vi "WMS_DSP_System.vi"() -> ()   [LabVIEW 2019]
uses:
  <vilib>/Analysis/baseanly.llb/IIR Cascade Filter (DBL).vi
  <vilib>/Analysis/Matrix/Numeric/Conversions/Array To Matrix - RA.vi
  <vilib>/Utility/file.llb/Write Delimited Spreadsheet (DBL).vi
  <vilib>/Utility/file.llb/Read Delimited Spreadsheet (DBL).vi
  <vilib>/measure/NI_MABase.lvlib
  <vilib>/Analysis/NI_AALPro.lvlib
  <vilib>/Analysis/NI_AALBase.lvlib
  <vilib>/Analysis/Matrix/NI_Matrix.lvlib
  <vilib>/gmath/NI_Gmath.lvlib
panel:
  in  "STOP":bool
  in  "stop":bool
  in  "?":T1(tab)
  in  "?":T2(tab)
  out "2f/1f":cluster{dbl[], dbl[]}(graph)
  out "I_OUT":cluster{dbl[], dbl[]}(graph)
  out "First derivative":cluster{dbl[], dbl[]}(graph)
  out "Second derivative":cluster{dbl[], dbl[]}(graph)
  out "FFT of 1f":cluster{"f0":dbl, "df":dbl, "magnitude":dbl[]}(graph)
  out "FFT of 2f":cluster{"f0":dbl, "df":dbl, "magnitude":dbl[]}(graph)
  out "Charakterystyki absorpcyjne":cluster{dbl[], dbl[]}[](graph)
  in  "c [ppmv]":dbl=1.7
  in  "Load data from file":bool
  in  "Data path":path
  in  "l [m]":dbl=1000.0
  in  "c2 [ppmv]":dbl=7750.0
  in  "l2 [m]":dbl=1000.0
  in  "FWHM [nm]":dbl
  in  "ddelta_di [nm/mA]":dbl
  in  "dlambda [nm]":dbl
  in  "P0 [mW]":dbl
  in  "dP_di [mW/mA]":dbl
  in  "i_bias [mA]":dbl
  in  "Phase_IM_FM [rad]":dbl
  in  "lambda0 [nm]":dbl
  in  "m":dbl
  in  "f_ramp [Hz]":dbl
  in  "f [Hz]":dbl
  in  "Zapis parametrów do pliku":bool
  in  "Odczyt parametrów z pliku":bool
  in  "START":bool
  in  "l_s [m]":dbl=1.0
  in  "c_s [ppmv]":dbl=1.0
  in  "l_S2 [m]":dbl=1.0
  in  "c_s2 [ppmv]":dbl=1.0
  in  "f_LP1":dbl=800.0
  in  "f_LP2":dbl=1600.0
  in  "K":dbl=100.0
  in  "R":dbl=50.0
  in  "?":T3(tab)
  out "Signal from CH1":waveform(dbl)(graph)
  out "Signal from CH2":waveform(dbl)(graph)
  out "Signal 2f/1f":waveform(dbl)(graph)
  out "Averaged signal 2f/1f":waveform(dbl)(graph)
  out "1f":waveform(dbl)(graph)
  out "2f":waveform(dbl)(graph)
  in  "DAQ":bool
  in  "Liczba usrednien":dbl=10.0
  out "Licznik usrednien":dbl
  in  "f_LP2_DAQ":dbl=1600.0 format="%0.3f"
  in  "f_LP1_DAQ":dbl=800.0 format="%0.3f"
  in  "f_prob":dbl=100000.0
  in  "f_ref":dbl=10000.0
  in  "?":enum32{"Fitting", "2f/1f sym", "2f/1f pom"}(tab)
  out "Fitting":cluster{"t1":dbl[], "yi":dbl[]}[](graph)
  out "Simulation":waveform(dbl)(graph)
  out "Measurment":waveform(dbl)(graph)
  in  "START":bool
  out "c [ppmv]":dbl
  out "SE":dbl
  out "Searching":dbl(knob) scale=0.0..10.0
  out "Concentration":dbl(knob) scale=0.0..10.0
  in  "c1 [ppmv]":dbl
  in  "c2 [ppmv]":dbl=10.0
  out "c_po":dbl
  out "SE2":dbl
  in  "Precisiion [ppmv]":dbl=0.1
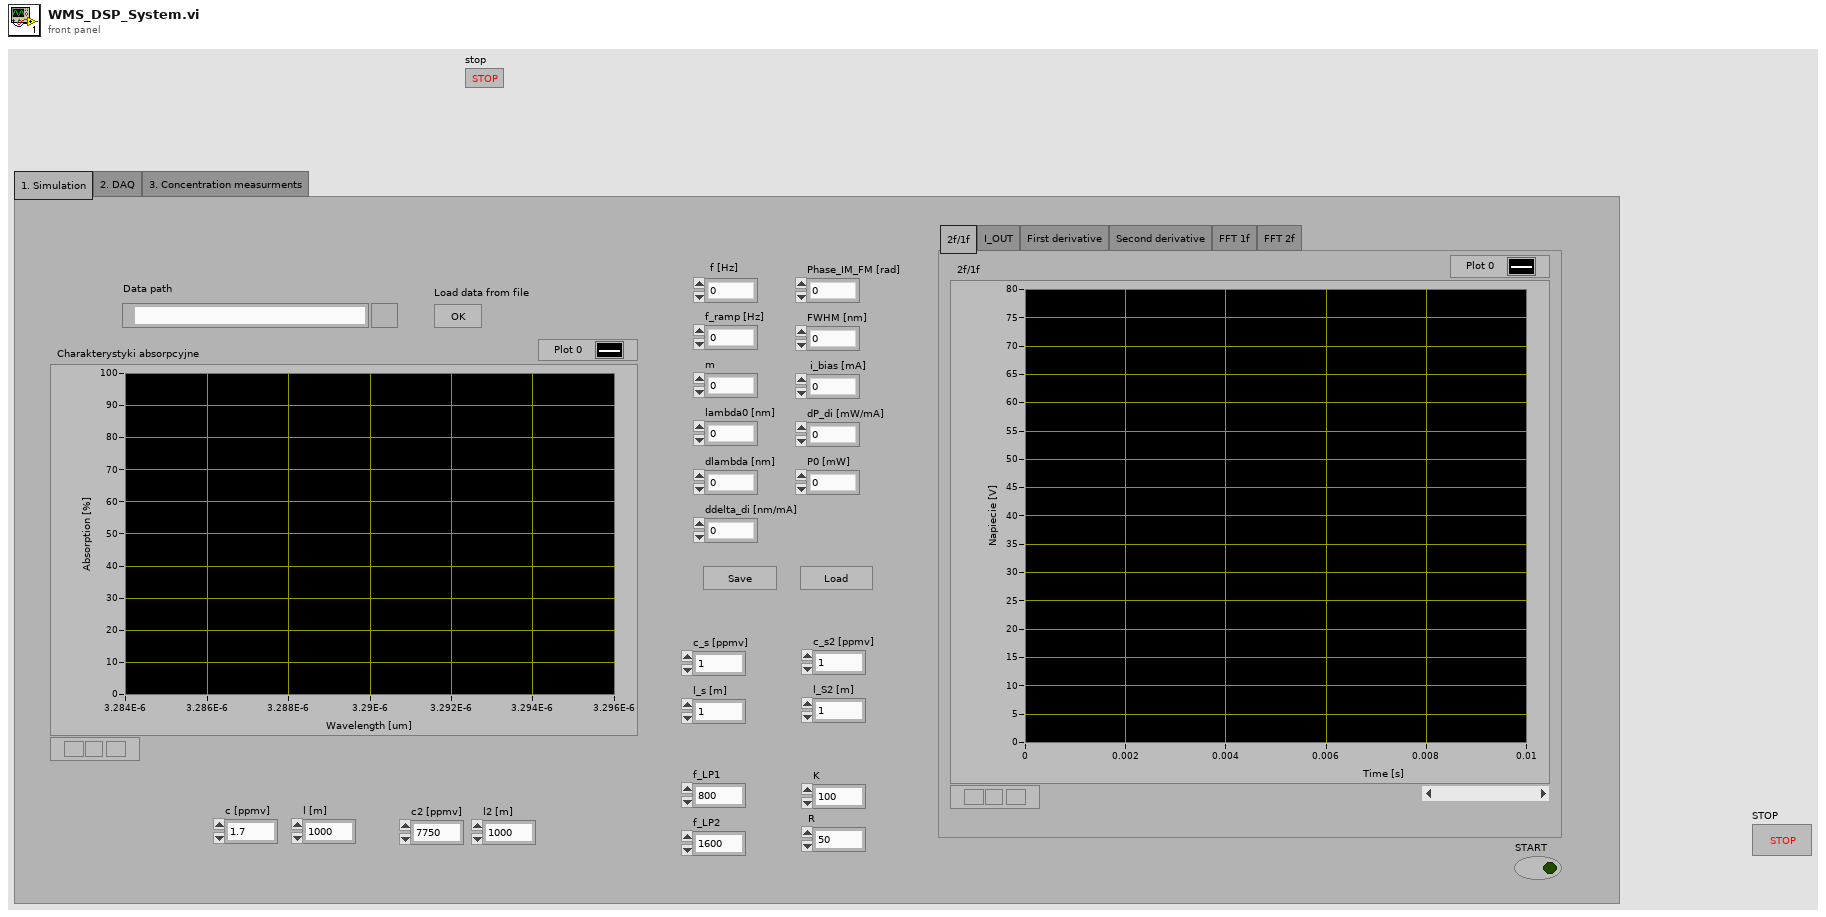
[diagram p1: front panel]
types:
  T1 = enum32{"1. Simulation", "2. DAQ", "3. Concentration measurments"}
  T2 = enum32{"2f/1f", "I_OUT", "First derivative", "Second derivative", "FFT 1f", "FFT 2f"}
  T3 = enum32{"Tor nr 1", "Tor nr 2", "2f/1f", "2f/1f usr", "1f me", "2f me"}
  T4 = cluster{"filter structure":enum32{"IIR 2nd Order", "IIR 4th Order"}, "Reverse Coefficients":dbl[], "Forward Coefficients":dbl[]}
  T5 = typedef "NI_Matrix.lvlib/RealMatrix.ctl" = dbl[][]
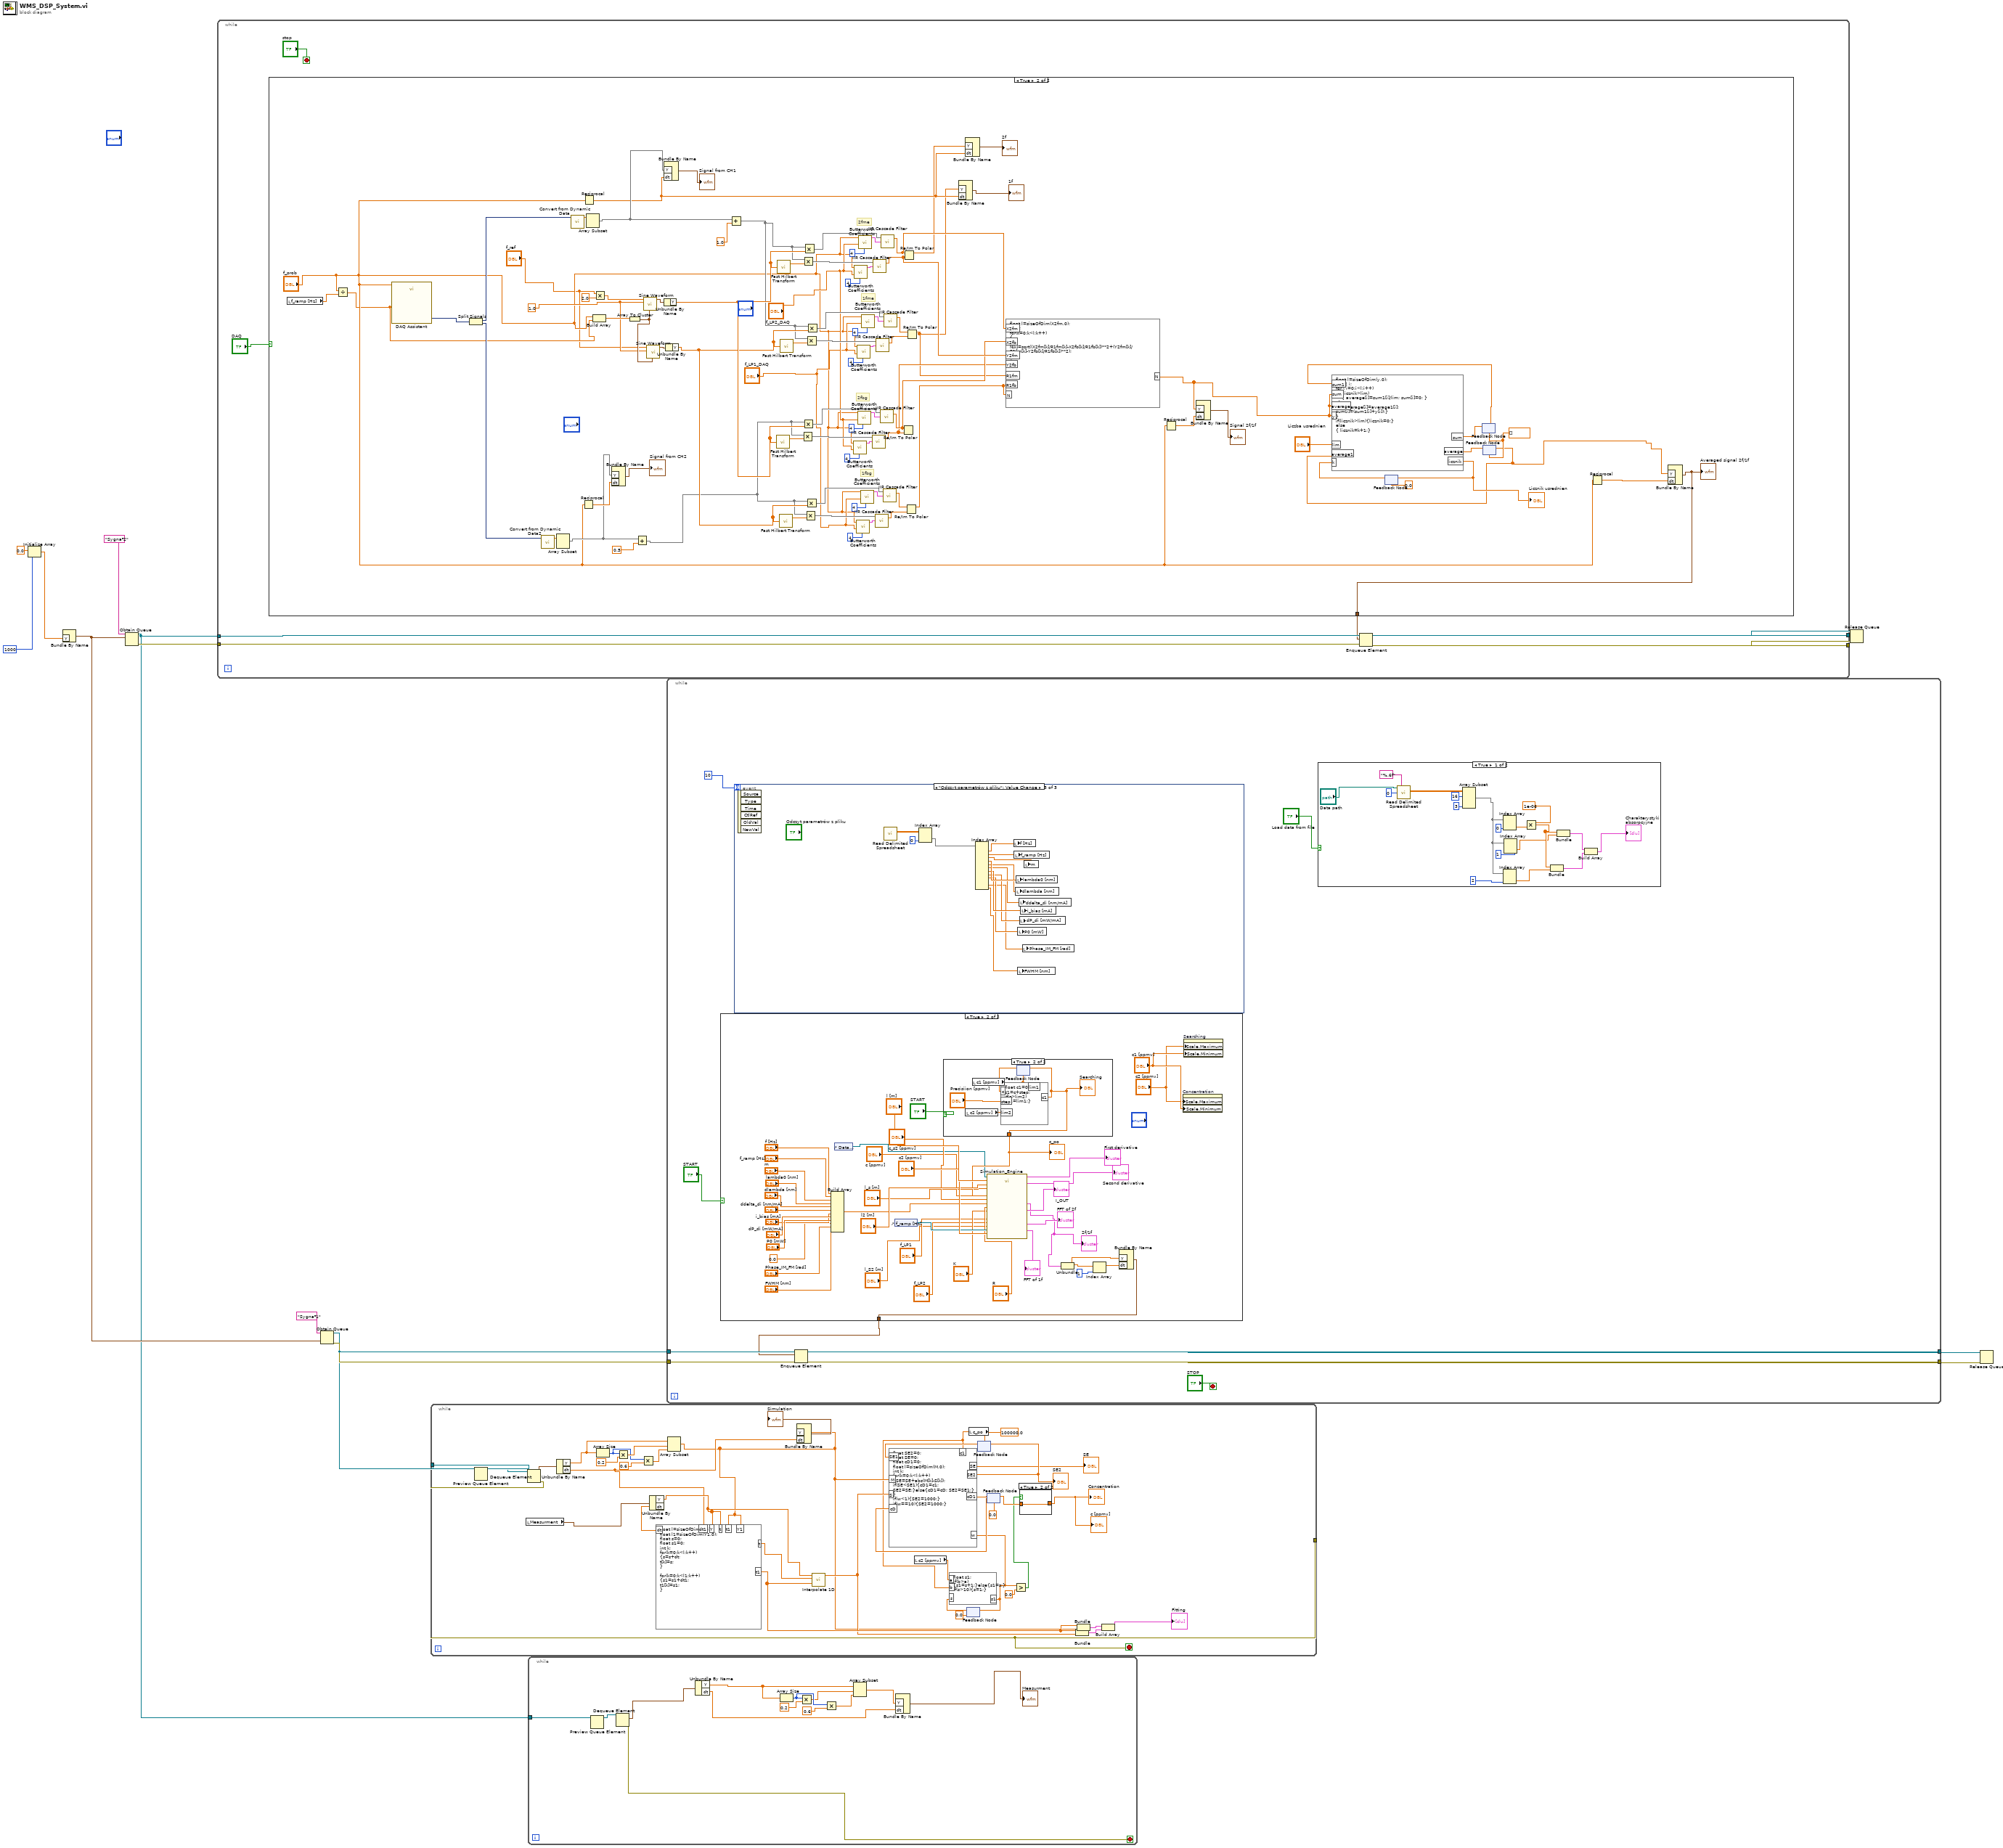
[diagram p0: block diagram]
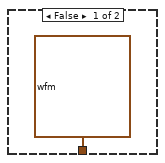
[diagram p2: hidden frame]
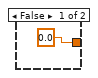
[diagram p3: hidden frame]
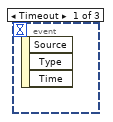
[diagram p5: hidden frame]
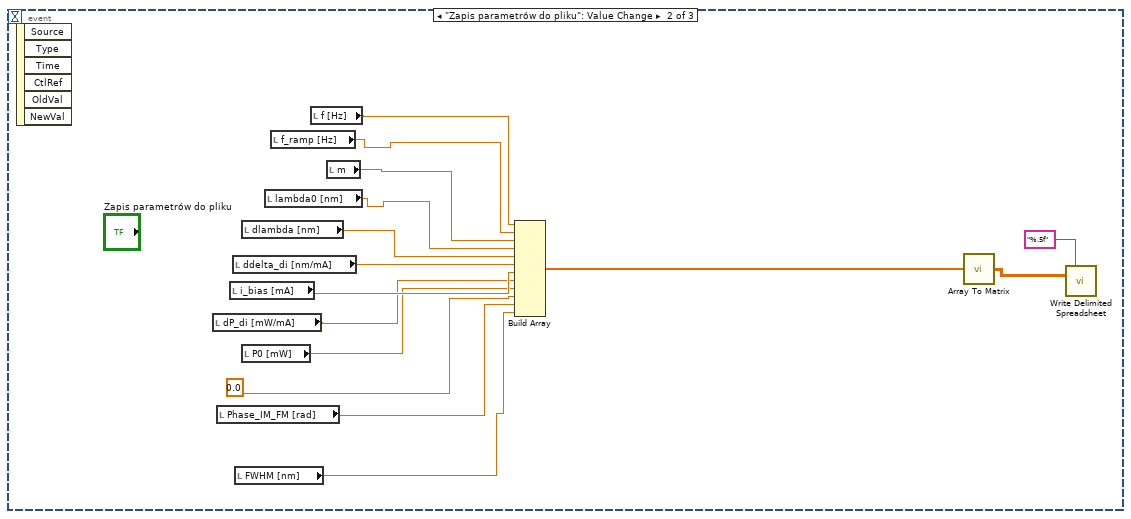
[diagram p6: hidden frame]
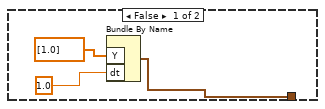
[diagram p7: hidden frame]
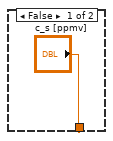
[diagram p8: hidden frame]
diagram:
  n1 = Initialize Array(0.0 ("element"), 1000 ("dimension size")) -> (w7:dbl[])
  n2 = Bundle By Name("Y"=w7) -> (w6:waveform(dbl))  [unwired: 1 in]
  n3 = Obtain Queue(name (unnamed)="Sygna³2", element data type=w6) -> (queue out=w1:refnum<queue>, error out=w5:errorcluster)  [unwired: 3 in, 1 out]
  n4 = while {
    tunnel: w1 -> [w20]
    tunnel: w5 -> [w19]
    tunnel: [w18] -> w4
    tunnel: [w17] -> w3
    stop <- "stop" stop-if-true
    n5 = case shown="True" "DAQ" {
      tunnel: [waveform(dbl) {"t0"=timestamp(0 s since 1904-01-01), "dt"=1.0, "Y"=[]} w36] -> w16
      frame False {
      }
      frame True {
        w46 = dbl[] [] ("y1")
        w86 = 1.0 ("amplitude")
        # "1fbg"
        # "2fbg"
        # "1fme"
        # "2fme"
        n6 = local read "f_ramp [Hz]"() -> (w26:dbl)
        n7 = Divide(x="f_prob", y=w26) -> (x/y=w24:dbl)
        n8 = call "DAQ Assistant"("rate"="f_prob", "number of samples"=w24) -> ("data"=w59:dynamicdata)  [unwired: 15 in, 2 out]
        n9 = Split Signals(w59) -> (w58:dynamicdata, w56:dynamicdata)  [unwired: 2 in]
        n10 = call "Convert from Dynamic Data2"("Dynamic Data Type"=w56) -> ("Array"=w55:dbl[])  [unwired: 3 in]
        n11 = Array Subset(array=w55) -> (w38:dbl[])  [unwired: 2 in]
        n12 = call "Convert from Dynamic Data"("Dynamic Data Type"=w58) -> ("Array"=w57:dbl[])  [unwired: 3 in]
        n13 = Reciprocal(x="f_prob") -> (1/x=w39:dbl)
        n14 = Reciprocal(x="f_prob") -> (1/x=w31:dbl)
        n15 = Array Subset(array=w57) -> (w40:dbl[])  [unwired: 2 in]
        n16 = Build Array("f_prob", w24) -> (w106:dbl[])
        n17 = Multiply(x="f_ref", y=2.0) -> (x*y=w87:dbl)
        n18 = Bundle By Name("Y"=w38, "dt"=w39) -> (→"Signal from CH2":waveform(dbl))  [unwired: 1 in]
        n19 = Array To Cluster(array=w106) -> (cluster=w98:cluster{"[0]":dbl, "[1]":dbl})
        n20 = Add(x=w38, y=0.5 ("high cutoff freq: fh")) -> (x+y=w53:dbl[])
        n21 = call <vilib>:"Sine Waveform.vi"("sampling info"=w98, "amplitude"=w86, "frequency"=w87) -> ("signal out"=w99:waveform(dbl))  [unwired: 7 in, 1 out]
        n22 = call <vilib>:"Sine Waveform.vi"("sampling info"=w98, "amplitude"=w86, "frequency"="f_ref") -> ("signal out"=w97:waveform(dbl))  [unwired: 7 in, 1 out]
        n23 = Unbundle By Name(w99) -> ("Y"=w69:dbl[])
        n24 = Bundle By Name("Y"=w40, "dt"=w31) -> (→"Signal from CH1":waveform(dbl))  [unwired: 1 in]
        n25 = Unbundle By Name(w97) -> ("Y"=w68:dbl[])
        n26 = Add(x=w40, y=1.0 ("high cutoff freq: fh")) -> (x+y=w54:dbl[])
        n27 = call <vilib>:"Fast Hilbert Transform.vi"("X"=w69) -> ("Hilbert{X}"=w84:dbl[])  [unwired: 1 out]
        n28 = call <vilib>:"Fast Hilbert Transform.vi"("X"=w69) -> ("Hilbert{X}"=w105:dbl[])  [unwired: 1 out]
        n29 = call <vilib>:"Fast Hilbert Transform.vi"("X"=w68) -> ("Hilbert{X}"=w78:dbl[])  [unwired: 1 out]
        n30 = call <vilib>:"Fast Hilbert Transform.vi"("X"=w68) -> ("Hilbert{X}"=w95:dbl[])  [unwired: 1 out]
        n31 = Multiply(x=w53, y=w84) -> (x*y=w79:dbl[])
        n32 = Multiply(x=w54, y=w105) -> (x*y=w100:dbl[])
        n33 = Multiply(x=w53, y=w69) -> (x*y=w66:dbl[])
        n34 = Multiply(x=w54, y=w69) -> (x*y=w67:dbl[])
        n35 = Multiply(x=w53, y=w78) -> (x*y=w71:dbl[])
        n36 = Multiply(x=w54, y=w95) -> (x*y=w89:dbl[])
        n37 = Multiply(x=w53, y=w68) -> (x*y=w75:dbl[])
        n38 = Multiply(x=w54, y=w68) -> (x*y=w92:dbl[])
        n39 = call <vilib>:"Butterworth Coefficients.vi"("order"=4, "low cutoff freq: fl"="f_LP2_DAQ", "sampling freq: fs"="f_prob") -> ("IIR Filter Cluster"=w80:T4)  [unwired: 7 in, 1 out]
        n40 = call <vilib>:"Butterworth Coefficients.vi"("order"=4, "low cutoff freq: fl"="f_LP2_DAQ", "sampling freq: fs"="f_prob") -> ("IIR Filter Cluster"=w101:T4)  [unwired: 7 in, 1 out]
        n41 = call <vilib>:"Butterworth Coefficients.vi"("order"=4, "low cutoff freq: fl"="f_LP1_DAQ", "sampling freq: fs"="f_prob") -> ("IIR Filter Cluster"=w72:T4)  [unwired: 7 in, 1 out]
        n42 = call <vilib>:"Butterworth Coefficients.vi"("order"=4, "low cutoff freq: fl"="f_LP1_DAQ", "sampling freq: fs"="f_prob") -> ("IIR Filter Cluster"=w90:T4)  [unwired: 7 in, 1 out]
        n43 = call <vilib>:"Butterworth Coefficients.vi"("order"=4, "low cutoff freq: fl"="f_LP2_DAQ", "sampling freq: fs"="f_prob") -> ("IIR Filter Cluster"=w81:T4)  [unwired: 7 in, 1 out]
        n44 = call <vilib>:"Butterworth Coefficients.vi"("order"=4, "low cutoff freq: fl"="f_LP2_DAQ", "sampling freq: fs"="f_prob") -> ("IIR Filter Cluster"=w102:T4)  [unwired: 7 in, 1 out]
        n45 = call <vilib>:"Butterworth Coefficients.vi"("order"=4, "low cutoff freq: fl"="f_LP1_DAQ", "sampling freq: fs"="f_prob") -> ("IIR Filter Cluster"=w74:T4)  [unwired: 7 in, 1 out]
        n46 = call <vilib>:"Butterworth Coefficients.vi"("order"=4, "low cutoff freq: fl"="f_LP1_DAQ", "sampling freq: fs"="f_prob") -> ("IIR Filter Cluster"=w91:T4)  [unwired: 7 in, 1 out]
        n47 = call-poly <vilib>:"IIR Cascade Filter.vi"("IIR Filter Cluster"=w80, "X"=w79) -> ("Filtered X"=w62:dbl[])  [unwired: 1 in, 1 out]
        n48 = call-poly <vilib>:"IIR Cascade Filter.vi"("IIR Filter Cluster"=w101, "X"=w100) -> ("Filtered X"=w65:dbl[])  [unwired: 1 in, 1 out]
        n49 = call-poly <vilib>:"IIR Cascade Filter.vi"("IIR Filter Cluster"=w72, "X"=w71) -> ("Filtered X"=w70:dbl[])  [unwired: 1 in, 1 out]
        n50 = call-poly <vilib>:"IIR Cascade Filter.vi"("IIR Filter Cluster"=w90, "X"=w89) -> ("Filtered X"=w88:dbl[])  [unwired: 1 in, 1 out]
        n51 = call-poly <vilib>:"IIR Cascade Filter.vi"("IIR Filter Cluster"=w81, "X"=w66) -> ("Filtered X"=w63:dbl[])  [unwired: 1 in, 1 out]
        n52 = call-poly <vilib>:"IIR Cascade Filter.vi"("IIR Filter Cluster"=w102, "X"=w67) -> ("Filtered X"=w64:dbl[])  [unwired: 1 in, 1 out]
        n53 = call-poly <vilib>:"IIR Cascade Filter.vi"("IIR Filter Cluster"=w74, "X"=w75) -> ("Filtered X"=w73:dbl[])  [unwired: 1 in, 1 out]
        n54 = call-poly <vilib>:"IIR Cascade Filter.vi"("IIR Filter Cluster"=w91, "X"=w92) -> ("Filtered X"=w61:dbl[])  [unwired: 1 in, 1 out]
        n55 = Re/Im To Polar(2:w62, 3:w63) -> ()  [unwired: 2 out]
        n56 = Re/Im To Polar(2:w65, 3:w64) -> (1:w30:dbl[])  [unwired: 1 out]
        n57 = Re/Im To Polar(2:w70, 3:w73) -> (1:w60:dbl[])  [unwired: 1 out]
        n58 = Re/Im To Polar(2:w88, 3:w61) -> (1:w28:dbl[])  [unwired: 1 out]
        n59 = Bundle By Name("Y"=w28, "dt"=w31) -> (→"1f":waveform(dbl))  [unwired: 1 in]
        n60 = Bundle By Name("Y"=w30, "dt"=w31) -> (→"2f":waveform(dbl))  [unwired: 1 in]
        n61 = formula code="float l=sizeOfDim(X2fm,0);\nint k;\nfor(k=0;k<l;k++)\n{\n\nN[k]=sqrt((X2fm[k]/R1fm[k]-X2fb[k]/R1fb[k])**2+(Y2fm[k]/R1fm[k]-Y2fb[k]/R1fb[k])**2);\n\n}"("X2fm"=w64, "X2fb"=w63, "Y2fm"=w65, "Y2fb"=w62, "R1fm"=w28, "R1fb"=w60, "N"=w60) -> ("N"=w43:dbl[])
        n62 = Reciprocal(x="f_prob") -> (1/x=w44:dbl)
        n63 = Bundle By Name("Y"=w43, "dt"=w44) -> (→"Signal 2f/1f":waveform(dbl))  [unwired: 1 in]
        n64 = feedback #1(0.0 ("licznik")) -> (w52:dbl)
        n65 = feedback #2(w46) -> (w50:dbl[])
        n66 = feedback #3(w46) -> (w32:dbl[])
        n67 = formula code="float l=sizeOfDim(y,0);\nint32 i;\nfor ( i=0;i<l;i++)\n{if(licznik>lim)\n    { average[i]=sum1[i]/lim; sum[i]=0; }\nelse\n    {average[i]=average1[i];\nsum[i]=(sum1[i]+y[i]);}\n}\nif(licznik>lim){licznik=0;}\nelse\n{ licznik=k+1;}"("y"=w43, "sum1"=w50, "k"=w52, "lim"="Liczba usrednien", "average1"=w32, "average"=w43, "sum"=w43) -> ("sum"=w48:dbl[], "licznik"=w49:dbl, "average"=w47:dbl[])
        "Licznik usrednien" <- w49
        n68 = feedback-in #1(w49) -> ()
        n69 = feedback-in #2(w48) -> ()
        n70 = feedback-in #3(w47) -> ()
        n71 = Reciprocal(x="f_prob") -> (1/x=w33:dbl)
        n72 = Bundle By Name("Y"=w32, "dt"=w33) -> (w36:waveform(dbl))  [unwired: 1 in]
        "Averaged signal 2f/1f" <- w36
      }
    }
    n73 = Enqueue Element(queue=w20, element=w16, error in (no error)=w19) -> (queue out=w18:refnum<queue>, error out=w17:errorcluster)  [unwired: 1 in, 1 out]
  }
  n74 = Obtain Queue(name (unnamed)="Sygna³1", element data type=w6) -> (queue out=w2:refnum<queue>, error out=w12:errorcluster)  [unwired: 3 in, 1 out]
  n75 = while {
    tunnel: [w130] -> _
    tunnel: w2 -> [w132]
    stop <- w130 stop-if-true
    n76 = Preview Queue Element(queue=w132) -> (queue out=w131:refnum<queue>)  [unwired: 2 in, 3 out]
    n77 = local read "Measurment"() -> (w117:waveform(dbl))
    n78 = Dequeue Element(queue=w131) -> (element=w144:waveform(dbl), error out=w130:errorcluster)  [unwired: 2 in, 2 out]
    n79 = Unbundle By Name(w144) -> ("Y"=w127:dbl[], "dt"=w125:dbl)
    n80 = Array Size(array=w127) -> (size(s)=w141:i32)
    n81 = Multiply(x=w141, y=0.2 ("c_s [ppmv]")) -> (x*y=w142:dbl)
    n82 = Multiply(x=w141, y=0.6 ("c_s [ppmv]")) -> (x*y=w139:dbl)
    n83 = Unbundle By Name(w117) -> ("Y"=w128:dbl[], "dt"=w129:dbl)
    n84 = Array Subset(array=w127, index=w142, length=w139) -> (w118:dbl[])
    n85 = formula code="float l=sizeOfDim(Y,0);\nfloat l1=sizeOfDim(Y1,0);\nfloat s=0;\nfloat s1=0;\nint k;\nfor(k=0;k<l;k++)\n{s=s+dt;\nt[k]=s;\n}\n\nfor(k=0;k<l1;k++)\n{s1=s1+dt1;\nt1[k]=s1;\n}"("dt"=w129, "Y"=w128, "t"=w128, "t1"=w118, "Y1"=w118, "dt1"=w125) -> ("t"=w126:dbl[], "t1"=w120:dbl[])
    n86 = Bundle By Name("Y"=w118, "dt"=w125) -> (→"Simulation":waveform(dbl))  [unwired: 1 in]
    n87 = call <vilib>:"Interpolate 1D.vi"("xi"=w120, "X"=w126, "Y"=w128) -> ("yi"=w119:dbl[])  [unwired: 6 in, 2 out]
    n88 = local read "c2 [ppmv]"() -> (w111:dbl)
    n89 = feedback #4(0.0) -> (w115:dbl)
    n90 = local read "c_po"() -> (w110:dbl)
    n91 = formula code="float s1;\nif(b>a)\n{s1=s+1;}else{s1=s;}\nif(s>10){s=1;}"("a"=w111, "b"=w110, "s"=w115) -> ("s1"=w108:dbl)
    n92 = feedback-in #4(w108) -> ()
    n93 = feedback #5(100000.0) -> (w136:dbl)
    n94 = feedback #6(0.0 ("cD1")) -> (w116:dbl)
    n95 = formula code="float SE2=0;\nfloat SE=0;\nfloat cD1=0;\nfloat l=sizeOfDim(M,0);\nint k;\nfor(k=0;k<l;k++)\n{SE=SE+abs(M[k]-S[k]);\nif(SE<SE1){cD1=c1; SE2=SE;}else{cD1=cD; SE2=SE1;}\n}\nif(w<1){SE2=1000;}\nif(w==10){SE2=1000;}"("M"=w118, "S"=w119, "c1"=w110, "cD"=w116, "SE1"=w136, "w"=w108) -> ("SE2"=w134:dbl, "cD1"=w138:dbl, "SE"=→"SE":dbl)
    "SE2" <- w134
    n96 = feedback-in #5(w134) -> ()
    n97 = feedback-in #6(w138) -> ()
    n98 = Greater?(x=w108, y=0.0) -> (0:w113:bool)
    n99 = case shown="True" w113 {
      tunnel: [0.0 w146] -> w109
      tunnel: w116 -> [_ w146]
      frame False {
      }
      frame True {
      }
    }
    "Concentration" <- w109
    "c [ppmv]" <- w109
    n100 = Bundle("t1"=w120, "yi"=w119) -> (w123:cluster{"t1":dbl[], "yi":dbl[]})  [unwired: 1 in]
    n101 = Bundle("t1"=w120, w118) -> (w122:cluster{"t1":dbl[], dbl[]})  [unwired: 1 in]
    n102 = Build Array(w122, w123) -> (→"Fitting":cluster{"t1":dbl[], "yi":dbl[]}[])
  }
  n103 = while {
    tunnel: w1 -> [w158]
    stop <- w151 stop-if-true
    n104 = Preview Queue Element(queue=w158) -> (queue out=w159:refnum<queue>)  [unwired: 2 in, 3 out]
    n105 = Dequeue Element(queue=w159) -> (element=w150:waveform(dbl), error out=w151:errorcluster)  [unwired: 2 in, 2 out]
    n106 = Unbundle By Name(w150) -> ("Y"=w147:dbl[], "dt"=w149:dbl)
    n107 = Array Size(array=w147) -> (size(s)=w156:i32)
    n108 = Multiply(x=w156, y=0.2 ("c_s [ppmv]")) -> (x*y=w155:dbl)
    n109 = Multiply(x=w156, y=0.6 ("c_s [ppmv]")) -> (x*y=w157:dbl)
    n110 = Array Subset(array=w147, index=w155, length=w157) -> (w148:dbl[])
    n111 = Bundle By Name("Y"=w148, "dt"=w149) -> (→"Measurment":waveform(dbl))  [unwired: 1 in]
  }
  n112 = while {
    tunnel: w2 -> [w168]
    tunnel: [w167] -> w13
    tunnel: w12 -> [w166]
    tunnel: [w165] -> w11
    stop <- "STOP" stop-if-true
    n113 = case shown="True" "START" {
      tunnel: [w216 w240] -> w163
      frame False {
        n114 = Bundle By Name("Y"=dbl[] [1.0], "dt"=1.0) -> (w216:waveform(dbl))  [unwired: 1 in]
      }
      frame True {
        n115 = Build Array("f [Hz]", "f_ramp [Hz]", "m", "lambda0 [nm]", "dlambda [nm]", "ddelta_di [nm/mA]", "i_bias [mA]", "dP_di [mW/mA]", "P0 [mW]", 0.0 ("element"), "Phase_IM_FM [rad]", "FWHM [nm]") -> (w236:dbl[])
        n116 = control-ref of="Data path"() -> (w235:refnum<vi>)
        n117 = control-ref of="f_ramp [Hz]"() -> (w234:refnum<vi>)
        n118 = case shown="True" "START" {
          tunnel: ["c_s [ppmv]" w264] -> w238
          frame False {
          }
          frame True {
            n119 = local read "c2 [ppmv]"() -> (w263:dbl)
            n120 = local read "c1 [ppmv]"() -> (w262:dbl)
            n121 = feedback #7(w262) -> (w265:dbl)
            n122 = formula code="float c1=0;\nc1=c+step;\nif(c>lim2)\n{c1=lim1;}"("c"=w265, "lim2"=w263, "lim1"=w262, "step"="Precisiion [ppmv]") -> ("c1"=w264:dbl)
            "Searching" <- w264
            n123 = feedback-in #7(w264) -> ()
          }
        }
        "c_po" <- w238
        n124 = call "Simulation_Engine.vi"("Path in"=w235, "c_s2 [ppmv]"="c_s2 [ppmv]", "l2 [m]"="l2 [m]", "l_s [m]"="l_s [m]", "c_s [ppmv]"=w238, "c [ppmv]"="c [ppmv]", "l [m]"="l [m]", "c2 [ppmv]"="c2 [ppmv]", "Array in"=w236, "reference in"=w234, "R"="R", "l_S2 [m]"="l_S2 [m]", "K"="K", "f_LP1"="f_LP1", "f_LP2"="f_LP2") -> ("I_OUT"=→"I_OUT":cluster{dbl[], dbl[]}, "Widmo drugiej pochodnej"=→"FFT of 2f":cluster{"f0":dbl, "df":dbl, "magnitude":dbl[]}, "Widmo pierwszej pochodnej"=→"FFT of 1f":cluster{"f0":dbl, "df":dbl, "magnitude":dbl[]}, "Pierwsza pochodna"=→"First derivative":cluster{dbl[], dbl[]}, "Druga pochodna"=→"Second derivative":cluster{dbl[], dbl[]}, "2f/1f"=w219:cluster{dbl[], dbl[]})  [unwired: 4 in, 3 out]
        "2f/1f" <- w219
        n125 = Unbundle(w219) -> (w242:dbl[], w237:dbl[])
        n126 = Index Array(array=w242, index=1) -> (element=w233:dbl)
        n127 = Bundle By Name("Y"=w237, "dt"=w233) -> (w240:waveform(dbl))  [unwired: 1 in]
        n128 = property on="Concentration" class="Knob (strict)"("Scale.Maximum"="c2 [ppmv]", "Scale.Minimum"="c1 [ppmv]") -> ()  [unwired: 2 in, 2 out]
        n129 = property on="Searching" class="Knob (strict)"("Scale.Maximum"="c2 [ppmv]", "Scale.Minimum"="c1 [ppmv]") -> ()  [unwired: 2 in, 2 out]
      }
    }
    n130 = event shown="[2] \"Odczyt parametrów z pliku\": Value Change" {
      selector: _ -> [_ _ _]
      dyn-events: _ -> [_ _ _]
      timeout: 10 -> [_ _ _]
      event Timeout {
        n131 = event-data() -> ()  [unwired: 1 in, 3 out]
      }
      event "Zapis parametrów do pliku": Value Change {
        n132 = event-data() -> ()  [unwired: 1 in, 6 out]
        n133 = local read "dP_di [mW/mA]"() -> (w191:dbl)
        n134 = local read "Phase_IM_FM [rad]"() -> (w189:dbl)
        n135 = local read "i_bias [mA]"() -> (w192:dbl)
        n136 = local read "ddelta_di [nm/mA]"() -> (w193:dbl)
        n137 = local read "FWHM [nm]"() -> (w187:dbl)
        n138 = local read "dlambda [nm]"() -> (w194:dbl)
        n139 = local read "P0 [mW]"() -> (w190:dbl)
        n140 = local read "lambda0 [nm]"() -> (w195:dbl)
        n141 = local read "f_ramp [Hz]"() -> (w197:dbl)
        n142 = local read "f [Hz]"() -> (w198:dbl)
        n143 = local read "m"() -> (w196:dbl)
        n144 = Build Array(w198, w197, w196, w195, w194, w193, w192, w191, w190, 0.0 ("element"), w189, w187) -> (w199:dbl[])
        n145 = call-poly <vilib>:"Array To Matrix.vi"("Real 1D Array"=w199) -> ("Real Matrix (Column Vector)"=w201:T5)
        n146 = call-poly <vilib>:"Write Delimited Spreadsheet.vi"("format (%.3f)"="%.5f", "2D data"=w201) -> ()  [unwired: 12 in, 2 out]
      }
      event "Odczyt parametrów z pliku": Value Change {
        n147 = event-data() -> ()  [unwired: 1 in, 6 out]
        n148 = call-poly <vilib>:"Read Delimited Spreadsheet.vi"() -> ("all rows"=w214:dbl[][])  [unwired: 10 in, 5 out]
        n149 = Index Array(array=w214, index (col)=0 ("disabled index (col)")) -> (element=w215:dbl[])  [unwired: 1 in]
        n150 = Index Array(array=w215) -> (element #1=w212:dbl, element #2=w211:dbl, element #3=w210:dbl, element #4=w209:dbl, element #5=w208:dbl, element #6=w207:dbl, element #7=w206:dbl, element #8=w205:dbl, element #9=w204:dbl, element #11=w203:dbl, element #12=w202:dbl)  [unwired: 12 in, 1 out]
        n151 = local write "f [Hz]"(w212) -> ()
        n152 = local write "f_ramp [Hz]"(w211) -> ()
        n153 = local write "dlambda [nm]"(w208) -> ()
        n154 = local write "lambda0 [nm]"(w209) -> ()
        n155 = local write "P0 [mW]"(w204) -> ()
        n156 = local write "FWHM [nm]"(w202) -> ()
        n157 = local write "ddelta_di [nm/mA]"(w207) -> ()
        n158 = local write "dP_di [mW/mA]"(w205) -> ()
        n159 = local write "i_bias [mA]"(w206) -> ()
        n160 = local write "Phase_IM_FM [rad]"(w203) -> ()
        n161 = local write "m"(w210) -> ()
      }
    }
    n162 = Enqueue Element(queue=w168, element=w163, error in (no error)=w166) -> (queue out=w167:refnum<queue>, error out=w165:errorcluster)  [unwired: 1 in, 1 out]
    n163 = case shown="True" "Load data from file" {
      frame True {
        n164 = call-poly <vilib>:"Read Delimited Spreadsheet.vi"("file path (dialog if empty)"="Data path", "format (%.3f)"="%.6f", "start of read offset (chars.:0)"=0) -> ("all rows"=w181:dbl[][])  [unwired: 7 in, 5 out]
        n165 = Array Subset(array=w181, index (row)=16 ("index"), length (col)=3 ("length")) -> (w182:dbl[][])  [unwired: 2 in]
        n166 = Index Array(array=w182, index (col)=2 ("disabled index (col)")) -> (element=w186:dbl[])  [unwired: 1 in]
        n167 = Index Array(array=w182, index (col)=0 ("disabled index (col)")) -> (element=w179:dbl[])  [unwired: 1 in]
        n168 = Index Array(array=w182, index (col)=1 ("disabled index (col)")) -> (element=w184:dbl[])  [unwired: 1 in]
        n169 = Multiply(x=1e-06, y=w179) -> (x*y=w185:dbl[])
        n170 = Bundle(w185, w186) -> (w183:cluster{dbl[], dbl[]})  [unwired: 1 in]
        n171 = Bundle(w185, w184) -> (w180:cluster{dbl[], dbl[]})  [unwired: 1 in]
        n172 = Build Array(w180, w183) -> (→"Charakterystyki absorpcyjne":cluster{dbl[], dbl[]}[])
      }
      frame False {
      }
    }
  }
  n173 = Release Queue(queue=w4, error in (no error)=w3) -> ()  [unwired: 1 in, 3 out]
  n174 = Release Queue(queue=w13, error in (no error)=w11) -> ()  [unwired: 1 in, 3 out]
